vi "mes~产品进站.vi"(8 "error in (no error)":errorcluster caption="错误输入（无错误）", 11 "identification":string caption="identification:") -> (0 "error out":errorcluster caption="错误输出", 2 "进站成功":bool)   [LabVIEW 2015]
uses:
  ctl/SendproCommonInStation.ctl
  ctl/ReceiveproCommonInStation.ctl
  Global.vi
panel:
  in  "Headers":string[][](array[string])=[["Content-Type", "text/xml;charset=UTF-8"], ["SOAPAction", "\"http://tempuri.org/IUserRightVerifyServiceImpl/UserRightVerify\""], ["Connection", "Keep-Alive"], ["User-Agent", "Apache-HttpClient/4.1.1 (java 1.5)"]]
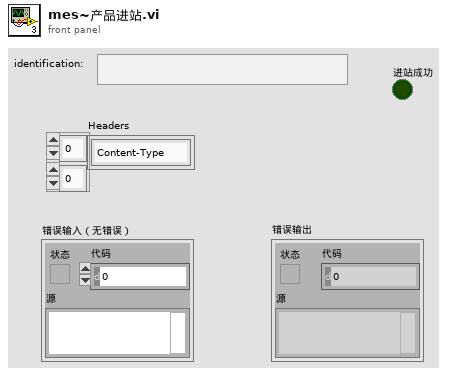
[diagram p1: front panel]
types:
  T1 = typedef "SendproCommonInStation.ctl" = cluster{"#attributes":cluster{"xmlns:soapenv":string, "xmlns:tem":string, "xmlns:cal":string}, "soapenv:Header":string, "soapenv:Body":cluster{"tem:ProCommon":cluster{"tem:model":cluster{"cal:equipNum":string, "cal:identification":string, "cal:productType":string, "cal:siteCode":string}}}}
  T2 = cluster{"接口地址(URL)":string, "设备编号(equipNum)":string, "站点名称(siteCode)":string, "生产类型(productType)":string, "试验单号(testOrderNum)":string}
  T3 = typedef "ReceiveproCommonInStation.ctl" = cluster{"#attributes":cluster{"xmlns:s":string}, "s:Body":cluster{"ProCommonResponse":cluster{"#attributes":cluster{"xmlns":string}, "ProCommonResult":cluster{"#attributes":cluster{"xmlns:a":string, "xmlns:i":string}, "a:ErrorCode":string, "a:ErrorMessage":string, "a:Success":string}}}}
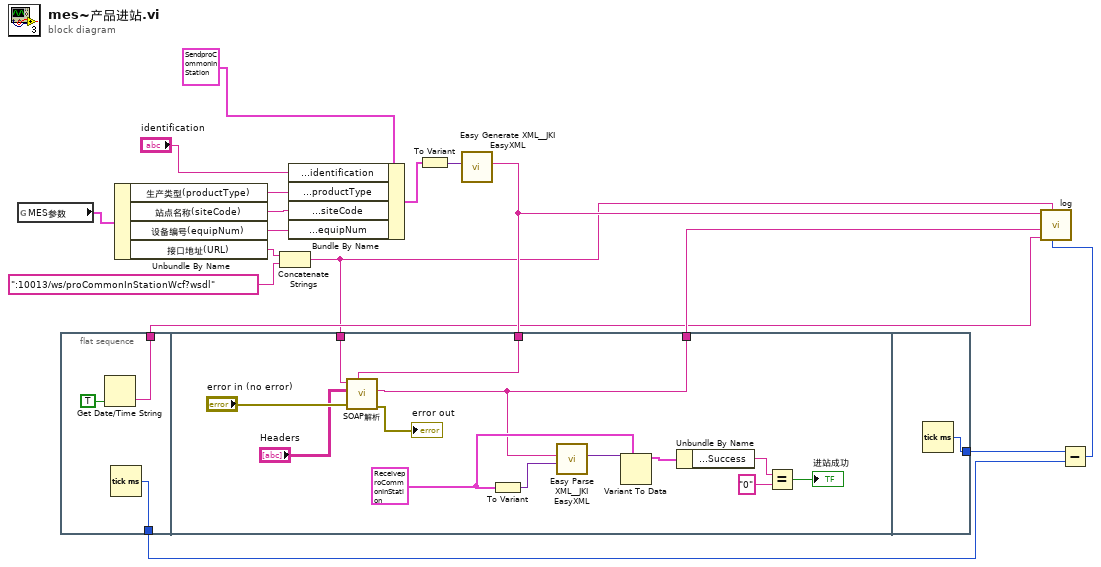
[diagram p0: block diagram]
diagram:
  n1 = global read "Global.vi" "MES参数"() -> (w13:T2)
  n2 = flat-sequence {
    tunnel: [w19] -> w6
    tunnel: [w18] -> w4
    tunnel: w8 -> [w23]
    tunnel: [w22] -> w7
    tunnel: w1 -> [w25]
    tunnel: [w34] -> w5
    frame #0 {
      n3 = Get Date/Time String(want seconds? (F)=TRUE ("需要秒？(F)")) -> (time string=w19:string)  [unwired: 2 in, 1 out]
      n4 = Tick Count (ms)() -> (millisecond timer value=w18:u32)
    }
    frame #1 {
      w27 = T3 {"#attributes"={"xmlns:s"="http://schemas.xmlsoap.org/soap/envelope/"}, "s:Body"={"ProCommonResponse"={"#attributes"={"xmlns"="http://tempuri.org/"}, "ProCommonResult"={"#attributes"={"xmlns:a"="http://schemas.datacontract.org/2004/07/EdgeUtility", "xmlns:i"="http://www.w3.org/2001/XMLSchema-instance"}, "a:ErrorCode"="", "a:ErrorMessage"="", "a:Success"=""}}}} ("s:Envelope")
      n5 = call "SOAP解析.vi"("DATA"=w23, "错误输入（无错误）"="error in (no error)", "Headers"="Headers", "URL"=w25) -> ("错误输出"=→"error out":errorcluster, "body"=w22:string)  [unwired: 5 in, 1 out]
      n6 = To Variant(anything=w27) -> (Variant=w33:variant)
      n7 = call <vilib>:"Easy Parse XML__JKI EasyXML.vi"("LabVIEW Data (Type)"=w33, "XML String"=w22) -> ("LabVIEW Data"=w32:variant)  [unwired: 8 in, 1 out]
      n8 = Variant To Data(type=w27, Variant=w32) -> (data=w31:T3)  [unwired: 1 in, 1 out]
      n9 = Unbundle By Name(w31) -> ("s:Body.ProCommonResponse.ProCommonResult.a:Success"=w30:string)
      n10 = Equal?(x=w30, y="0") -> (x = y?=→"进站成功":bool)
    }
    frame #2 {
      n11 = Tick Count (ms)() -> (millisecond timer value=w34:u32)
    }
  }
  n12 = Unbundle By Name(w13) -> ("生产类型(productType)"=w9:string, "站点名称(siteCode)"=w14:string, "设备编号(equipNum)"=w15:string, "接口地址(URL)"=w11:string)
  n13 = Concatenate Strings(w11, ":10013/ws/proCommonInStationWcf?wsdl") -> (w1:string)
  n14 = Bundle By Name(cluster=T1 {"#attributes"={"xmlns:soapenv"="http://schemas.xmlsoap.org/soap/envelope/", "xmlns:tem"="http://tempuri.org/", "xmlns:cal"="http://schemas.datacontract.org/2004/07/CalbProductCommonInStationService"}, "soapenv:Header"="", "soapenv:Body"={"tem:ProCommon"={"tem:model"={"cal:equipNum"="", "cal:identification"="", "cal:productType"="", "cal:siteCode"=""}}}} ("soapenv:Envelope"), "soapenv:Body.tem:ProCommon.tem:model.cal:identification"="identification", "soapenv:Body.tem:ProCommon.tem:model.cal:productType"=w9, "soapenv:Body.tem:ProCommon.tem:model.cal:siteCode"=w14, "soapenv:Body.tem:ProCommon.tem:model.cal:equipNum"=w15) -> (w17:T1)
  n15 = To Variant(anything=w17) -> (Variant=w16:variant)
  n16 = call <vilib>:"Easy Generate XML__JKI EasyXML.vi"("LabVIEW Data"=w16) -> ("XML String"=w8:string)  [unwired: 9 in, 1 out]
  n17 = Subtract(x=w5, y=w4) -> (x-y=w3:u32)
  n18 = call "log.vi"("接口耗时"=w3, "URL"=w1, "StartTime"=w6, "响应报文"=w7, "发送报文"=w8) -> ()  [unwired: 7 in]
